vi "Test.vi"   [LabVIEW 2019]
doc: "This VI is called when test mode begins, and will automatically be terminated when it ends. You can add manual or automatic tests and invoke them from the dashboard."
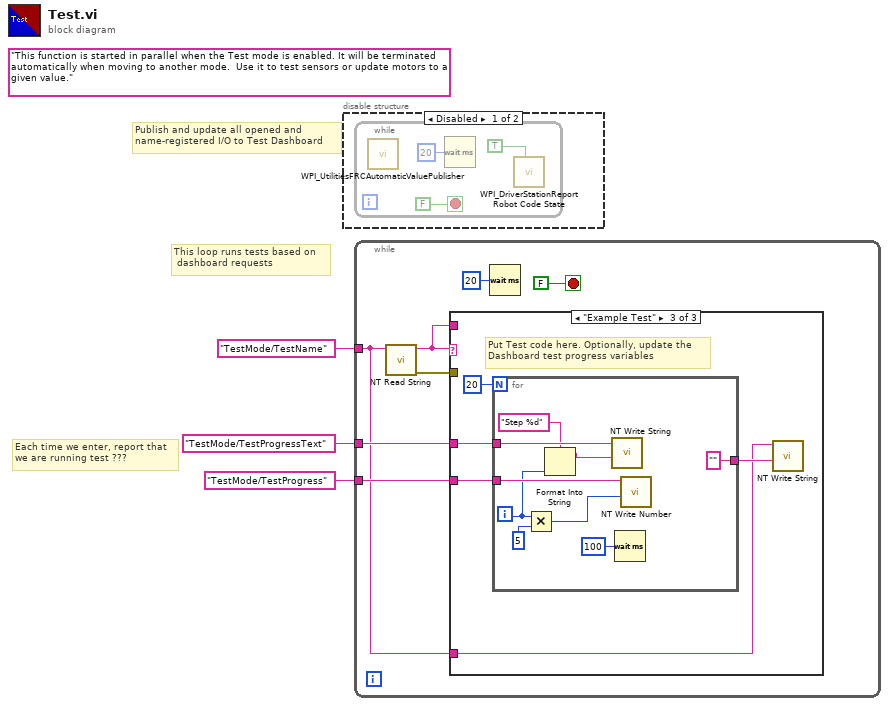
[diagram p0: block diagram]
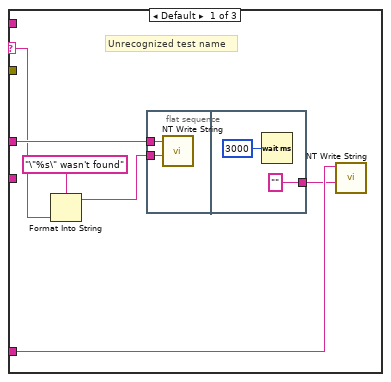
[diagram p3: hidden frame]
diagram:
  (unwired) "This function is started in parallel when the Test mode is enabled. It will be terminated automatically when moving to another mode.  Use it to test sensors or update motors to a given value."
  # "This loop runs tests based on \n dashboard requests"
  # "Publish and update all opened and\nname-registered I/O to Test Dashboard"
  # "Each time we enter, report that\nwe are running test ???"
  n1 = disable-structure shown="Disabled" {
    frame Disabled {
      n2 = while {
        stop <- FALSE stop-if-true
        n3 = call <vilib>:"WPI_UtilitiesFRCAutomaticValuePublisher.vi"() -> ()  [unwired: 12 in]
        n4 = Wait (ms)(milliseconds to wait=u32 20) -> ()  [unwired: 1 out]
        n5 = call <vilib>:"WPI_DriverStationReport Robot Code State.vi"("Test"=TRUE ("Autonomous")) -> ()  [unwired: 10 in, 1 out]
      }
    }
    frame Enabled {
    }
  }
  n6 = while {
    tunnel: "TestMode/TestName" ("Name") -> [w8]
    tunnel: "TestMode/TestProgressText" ("Name") -> [w11]
    tunnel: "TestMode/TestProgress" ("Name") -> [w10]
    stop <- FALSE stop-if-true
    n7 = call <vilib>:"NT Read String.vi"("Name"=w8) -> ("error out"=w7:errorcluster, "String"=w9:string)  [unwired: 9 in]
    n8 = case shown="\"Example Test\"" w9 {
      selector: w9 -> [w18 _ _]
      tunnel: w8 -> [w15 _ w24]
      tunnel: w11 -> [w19 _ w27]
      tunnel: w10 -> [_ _ w28]
      tunnel: w9 -> [_ _ _]
      tunnel: w7 -> [_ _ _]
      frame Default {
        # "Unrecognized test name"
        n9 = Format Into String(format string="\"%s\" wasn't found" ("Name"), w18) -> (resulting string=w17:string)  [unwired: 2 in, 1 out]
        n10 = flat-sequence {
          tunnel: w19 -> [w20]
          tunnel: w17 -> [w21]
          tunnel: ["" ("Name")] -> w14
          frame #0 {
            n11 = call <vilib>:"NT Write String.vi"("String"=w21, "Name"=w20) -> ()  [unwired: 9 in, 1 out]
          }
          frame #1 {
            n12 = Wait (ms)(milliseconds to wait=u32 3000) -> ()  [unwired: 1 out]
          }
        }
        n13 = call <vilib>:"NT Write String.vi"("String"=w14, "Name"=w15) -> ()  [unwired: 9 in, 1 out]
      }
      frame "" {
        # "No test to run"
      }
      frame "Example Test" {
        # "Put Test code here. Optionally, update the\nDashboard test progress variables"
        n14 = for {
          N: 20 -> [_]
          tunnel: w28 -> [w37]
          tunnel: w27 -> [w35]
          tunnel: ["" ("String")] -> w25
          i -> [w32]
          n15 = Multiply(x=w32, y=u32 5 ("milliseconds to wait")) -> (x*y=w33:u32)
          n16 = Format Into String(format string="Step %d", w32) -> (resulting string=w30:string)  [unwired: 2 in, 1 out]
          n17 = call <vilib>:"NT Write String.vi"("String"=w30, "Name"=w35) -> ()  [unwired: 9 in, 1 out]
          n18 = Wait (ms)(milliseconds to wait=u32 100) -> ()  [unwired: 1 out]
          n19 = call <vilib>:"NT Write Number.vi"("Numeric"=w33, "Name"=w37) -> ()  [unwired: 9 in, 1 out]
        }
        n20 = call <vilib>:"NT Write String.vi"("String"=w25, "Name"=w24) -> ()  [unwired: 9 in, 1 out]
      }
    }
    n21 = Wait (ms)(milliseconds to wait=u32 20) -> ()  [unwired: 1 out]
  }
